vi "Extract_to_JSON.vi"() -> ()   [LabVIEW 2019]
uses:
  a92b969b-4199-414a-85c5-08ca7c07869d.vi
  <vilib>/JDP Science/JSONtext/JSONtext.lvlib
panel:
  in  "Output":path
  in  "File":path
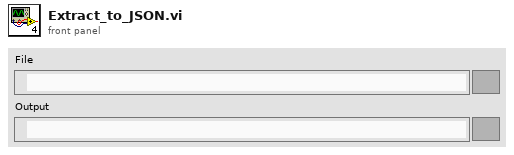
[diagram p1: front panel]
types:
  T1 = cluster{"f":dbl, "a2":dbl, "a1":dbl, "a8":dbl, "a4":dbl, "a7":dbl}
  T2 = enum16{"open", "replace", "create", "open or create", "replace or create", "replace or create with confirmation"}
  T3 = enum16{"open", "open or create", "create or replace", "create", "open (read-only)"}
  T4 = cluster{"x":dbl[], "y":dbl[], "z":dbl[], "t0":timestamp, "dt":dbl, "f":dbl}
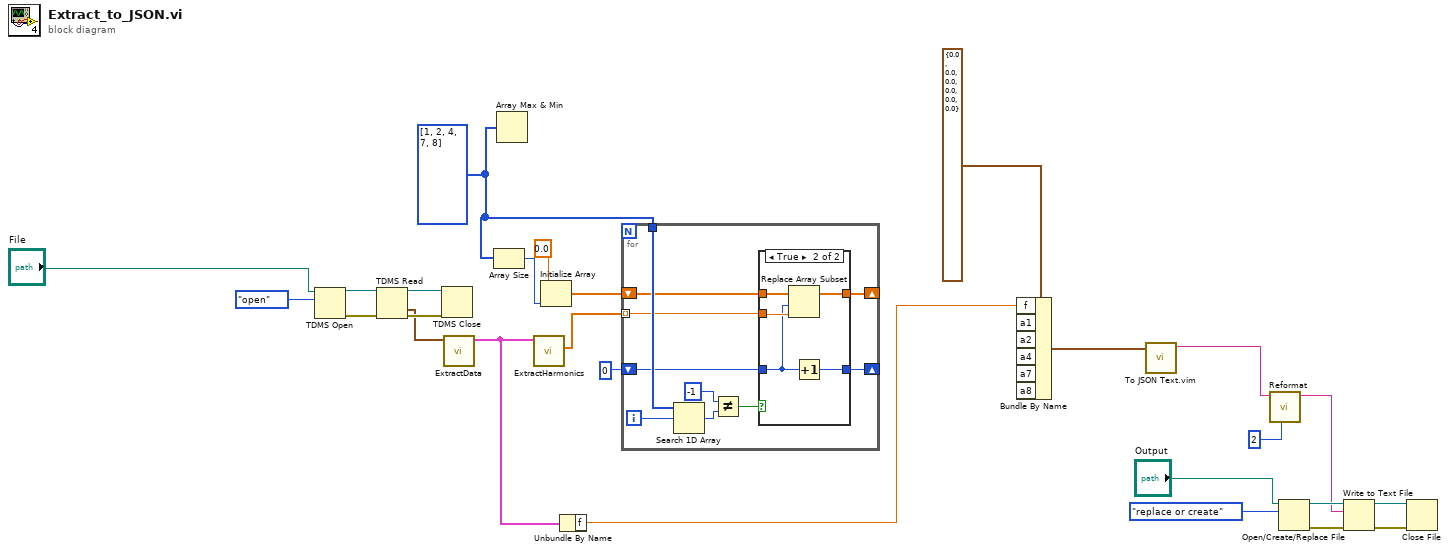
[diagram p0: block diagram]
diagram:
  w10 = i32[] [1, 2, 4, 7, 8] ("initialized array")
  n1 = TDMS Open(10:T3."open" ("operation (0:open)"), 11:"File") -> (0:w24:errorcluster, 3:w25:refnum<k34>)  [unwired: 5 in]
  n2 = TDMS Read(0:w25, 11:w24) -> (4:w23:refnum<k34>, 10:w21:waveform(dbl)[], 15:w22:errorcluster)  [unwired: 6 in, 3 out]
  n3 = TDMS Close(8:w22, 11:w23) -> ()  [unwired: 2 out]
  n4 = call "ExtractData.vi"("Data input"=w21) -> ("Data cluster"=w4:T4)  [unwired: 10 in]
  n5 = Array Size(array=w10) -> (size(s)=w9:i32)
  n6 = Array Max & Min(array=w10) -> ()  [unwired: 4 out]
  n7 = call "ExtractHarmonics.vi"("Input cluster"=w4) -> ("components level"=w7:dbl[])  [unwired: 9 in, 1 out]
  n8 = Initialize Array(0.0 ("element"), w9) -> (w13:dbl[])
  n9 = Unbundle By Name(w4) -> ("f"=w1:dbl)
  n10 = for {
    tunnel: w10 -> [w36]
    shift-right: [w30] -> _
    shift-left: w13 -> [w31]
    shift-right: [w28] -> _
    shift-left: 0 -> [w29]
    tunnel: w7 -> [w27] mode=indexing
    i -> [w35]
    n11 = Search 1D Array(1D array=w36, element=w35) -> (index of element=w34:i32)  [unwired: 1 in]
    n12 = Not Equal?(x=-1, y=w34) -> (x != y?=w32:bool)
    n13 = case shown="True" w32 {
      tunnel: w31 -> [w38 w42]
      tunnel: [w38 w43] -> w30
      tunnel: w27 -> [_ w41]
      tunnel: w29 -> [w37 w40]
      tunnel: [w37 w39] -> w28
      frame False {
      }
      frame True {
        n14 = Replace Array Subset(array=w42, new element=w41, index=w40) -> (w43:dbl[])
        n15 = Increment(x=w40) -> (x+1=w39:i32)
      }
    }
  }
  n16 = Bundle By Name(cluster=T1 {"f"=0.0, "a2"=0.0, "a1"=0.0, "a8"=0.0, "a4"=0.0, "a7"=0.0} ("input cluster"), "f"=w1) -> (w2:T1)  [unwired: 5 in]
  n17 = call "To JSON Text.vim"("Anything"=w2) -> ("<JSON>"=w8:string)  [unwired: 9 in, 1 out]
  n18 = call <vilib>:"Reformat.vi"("Pretty Print Levels"=2, "JSON"=w8) -> ("<JSON>First JSON Value\n\n<JSON>"=w15:string)  [unwired: 6 in, 3 out]
  n19 = Open/Create/Replace File(file path (use dialog)="Output", operation (0:open)=T2."replace or create") -> (refnum out=w18:refnum<file>, error out=w17:errorcluster)  [unwired: 4 in, 1 out]
  n20 = Write to Text File(file (use dialog)=w18, text=w15, error in=w17) -> (refnum out=w20:refnum<file>, error out=w19:errorcluster)  [unwired: 1 in, 1 out]
  n21 = Close File(refnum=w20, error in=w19) -> ()  [unwired: 2 out]
